vi "Base64AsValue.vi"(8 "error in":errorcluster, 11 "scalar value (binary string)":string) -> (0 "error out":errorcluster, 3 "scalar string":string)   [LabVIEW 2014]
doc: "Base64 encode a binary string and format it as an XML-RPC base64 type"
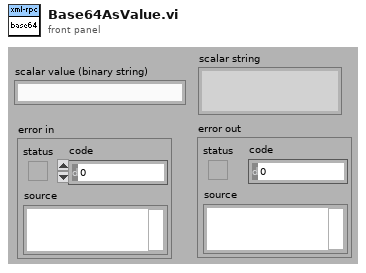
[diagram p1: front panel]
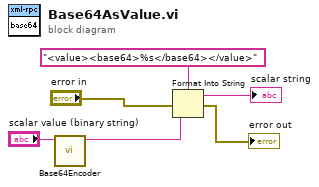
[diagram p0: block diagram]
diagram:
  n1 = call "Base64Encoder.vi"("String In"="scalar value (binary string)") -> ("String Out"=w1:string)  [unwired: 9 in, 1 out]
  n2 = Format Into String(format string="<value><base64>%s</base64></value>", error in="error in", w1) -> (resulting string=→"scalar string":string, error out=→"error out":errorcluster)  [unwired: 1 in]
